vi "Motors_Stop_Global.vi"(0 "error in":errorcluster caption="Fehler (Eingang, kein Fehler)") -> ()   [LabVIEW 2016]
uses:
  Utility/Global_Stage.vi
  Utility/Global Constants.vi
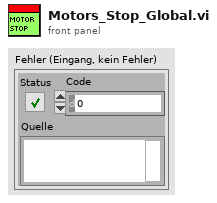
[diagram p1: front panel]
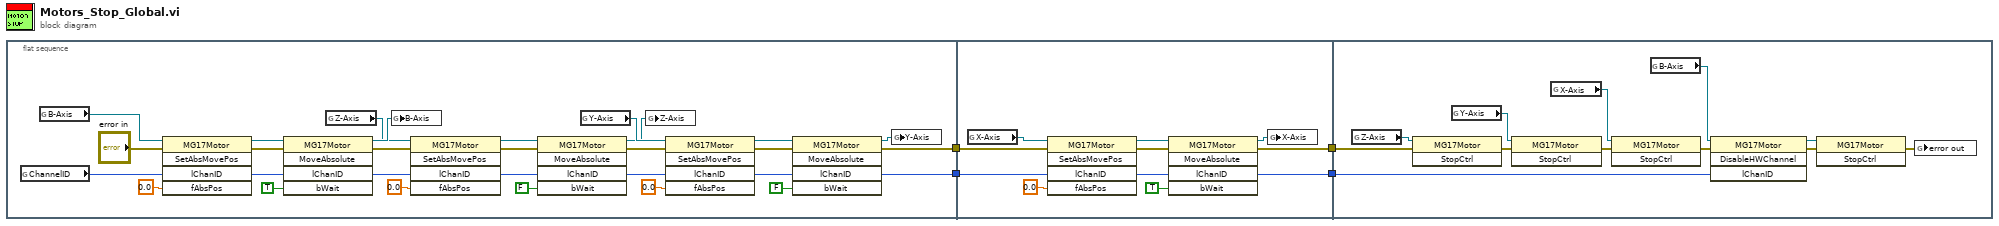
[diagram p0: block diagram]
diagram:
  n1 = flat-sequence {
    tunnel: [w27] -> w4
    tunnel: [w5] -> w3
    tunnel: w4 -> [w41]
    tunnel: w3 -> [w37]
    tunnel: [w35] -> w2
    tunnel: [w34] -> w1
    tunnel: w2 -> [w53]
    tunnel: w1 -> [w45]
    frame #0 {
      n2 = global read "Global_Stage.vi" "ChannelID"() -> (w16:i32)
      n3 = global read "Global_Stage.vi" "B-Axis"() -> (w24:refnum<k7>)
      n4 = invoke class="MG17Motor" method="SetAbsMovePos"(reference=w24, error in="error in", "lChanID"=w16, "fAbsPos"=sgl 0.0) -> (reference out=w23:refnum<k7>, error out=w9:errorcluster, "lChanID"=w15:i32)  [unwired: 1 in, 2 out]
      n5 = invoke class="MG17Motor" method="MoveAbsolute"(reference=w23, error in=w9, "lChanID"=w15, "bWait"=TRUE) -> (reference out=w22:refnum<k7>, error out=w8:errorcluster, "lChanID"=w14:i32)  [unwired: 1 in, 2 out]
      n6 = global read "Global_Stage.vi" "Z-Axis"() -> (w21:refnum<k7>)
      n7 = global write "Global_Stage.vi" "B-Axis"(w22) -> ()
      n8 = invoke class="MG17Motor" method="SetAbsMovePos"(reference=w21, error in=w8, "lChanID"=w14, "fAbsPos"=sgl 0.0) -> (reference out=w20:refnum<k7>, error out=w7:errorcluster, "lChanID"=w13:i32)  [unwired: 1 in, 2 out]
      n9 = invoke class="MG17Motor" method="MoveAbsolute"(reference=w20, error in=w7, "lChanID"=w13, "bWait"=FALSE) -> (reference out=w19:refnum<k7>, error out=w6:errorcluster, "lChanID"=w12:i32)  [unwired: 1 in, 2 out]
      n10 = global read "Global_Stage.vi" "Y-Axis"() -> (w33:refnum<k7>)
      n11 = global write "Global_Stage.vi" "Z-Axis"(w19) -> ()
      n12 = invoke class="MG17Motor" method="SetAbsMovePos"(reference=w33, error in=w6, "lChanID"=w12, "fAbsPos"=sgl 0.0) -> (reference out=w31:refnum<k7>, error out=w32:errorcluster, "lChanID"=w30:i32)  [unwired: 1 in, 2 out]
      n13 = invoke class="MG17Motor" method="MoveAbsolute"(reference=w31, error in=w32, "lChanID"=w30, "bWait"=FALSE) -> (reference out=w11:refnum<k7>, error out=w5:errorcluster, "lChanID"=w27:i32)  [unwired: 1 in, 2 out]
      n14 = global write "Global_Stage.vi" "Y-Axis"(w11) -> ()
    }
    frame #1 {
      n15 = global read "Global_Stage.vi" "X-Axis"() -> (w44:refnum<k7>)
      n16 = invoke class="MG17Motor" method="SetAbsMovePos"(reference=w44, error in=w37, "lChanID"=w41, "fAbsPos"=sgl 0.0) -> (reference out=w42:refnum<k7>, error out=w36:errorcluster, "lChanID"=w40:i32)  [unwired: 1 in, 2 out]
      n17 = invoke class="MG17Motor" method="MoveAbsolute"(reference=w42, error in=w36, "lChanID"=w40, "bWait"=TRUE) -> (reference out=w43:refnum<k7>, error out=w35:errorcluster, "lChanID"=w34:i32)  [unwired: 1 in, 2 out]
      n18 = global write "Global_Stage.vi" "X-Axis"(w43) -> ()
    }
    frame #2 {
      n19 = global read "Global_Stage.vi" "Z-Axis"() -> (w55:refnum<k7>)
      n20 = invoke class="MG17Motor" method="StopCtrl"(reference=w55, error in=w53) -> (error out=w52:errorcluster)  [unwired: 1 in, 2 out]
      n21 = global read "Global_Stage.vi" "Y-Axis"() -> (w54:refnum<k7>)
      n22 = invoke class="MG17Motor" method="StopCtrl"(reference=w54, error in=w52) -> (error out=w51:errorcluster)  [unwired: 1 in, 2 out]
      n23 = global read "Global_Stage.vi" "X-Axis"() -> (w56:refnum<k7>)
      n24 = invoke class="MG17Motor" method="StopCtrl"(reference=w56, error in=w51) -> (error out=w49:errorcluster)  [unwired: 1 in, 2 out]
      n25 = global read "Global_Stage.vi" "B-Axis"() -> (w47:refnum<k7>)
      n26 = invoke class="MG17Motor" method="DisableHWChannel"(reference=w47, error in=w49, "lChanID"=w45) -> (reference out=w50:refnum<k7>, error out=w48:errorcluster)  [unwired: 1 in, 2 out]
      n27 = invoke class="MG17Motor" method="StopCtrl"(reference=w50, error in=w48) -> (error out=w46:errorcluster)  [unwired: 1 in, 2 out]
      n28 = global write "Global Constants.vi" "error out"(w46) -> ()
    }
  }
